vi "NEW_PRN Generation_Station1.vi"(8 "error in (no error)":errorcluster, 11 "Cluster in":T2) -> (0 "error out":errorcluster, 2 "cluster out":T2, 3 "QR CODE":string)   [LabVIEW 2017]
uses:
  <vilib>/addons/database/Connection.llb/Conn ObjectReference.ctl
  <vilib>/addons/database/NI_Database_API.lvlib
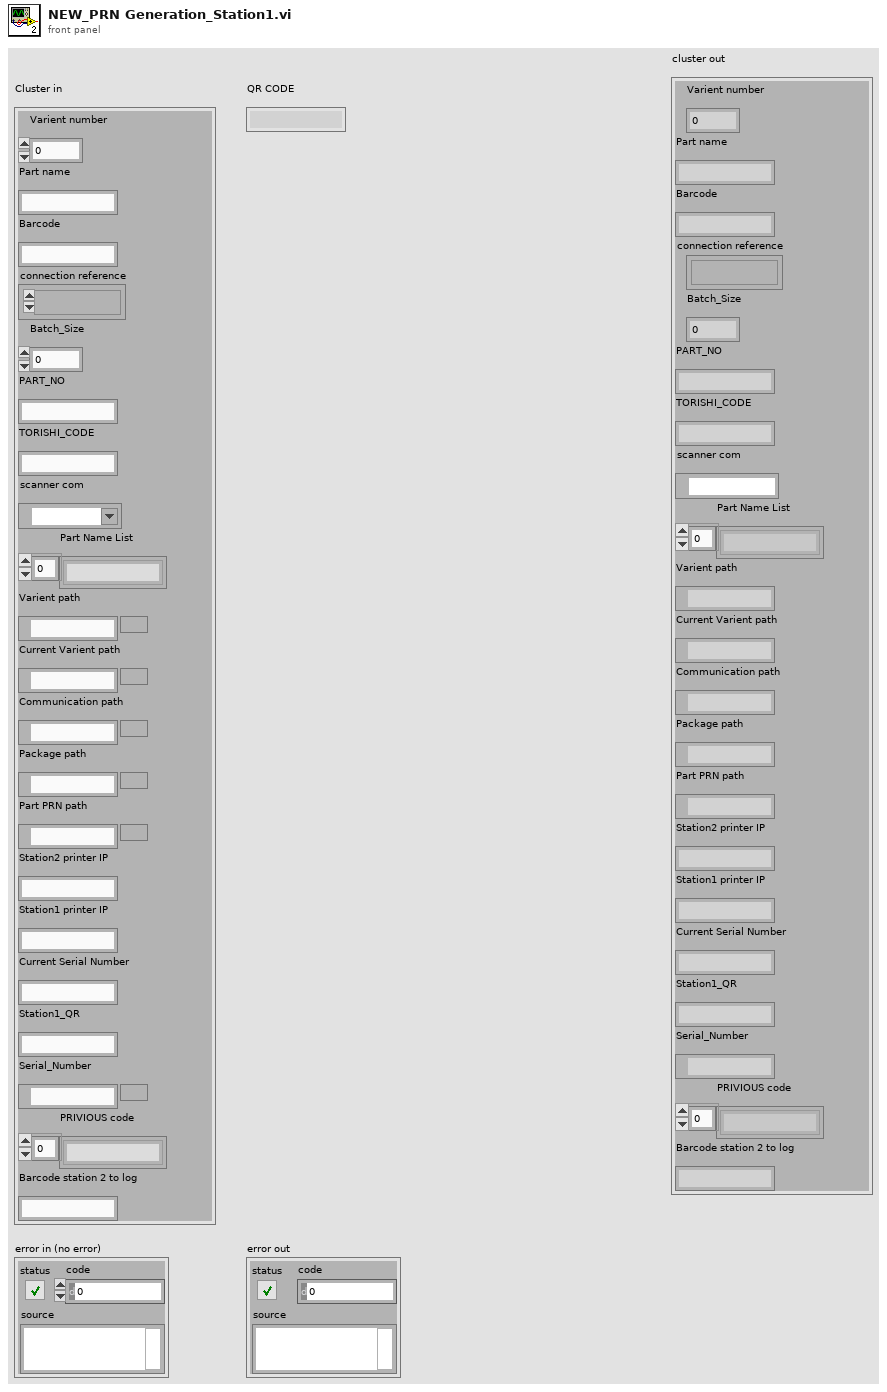
[diagram p1: front panel]
types:
  T1 = typedef "NI_Database_API.lvlib/Conn ObjectReference.ctl" = refnum<k1>
  T2 = cluster{"Varient number":u16, "Part name":string, "Barcode":string, "connection reference":T1, "Batch_Size":u16, "PART_NO":string, "TORISHI_CODE":string, "scanner com":refnum<visa-resource-name>, "Part Name List":string[], "Varient path":path, "Current Varient path":path, "Communication path":path, "Package path":path, "Part PRN path":path, "Station2 printer IP":string, "Station1 printer IP":string, "Current Serial Number":string, "Station1_QR":string, "Serial_Number":path, "PRIVIOUS code":string[], "Barcode station 2 to log":string}
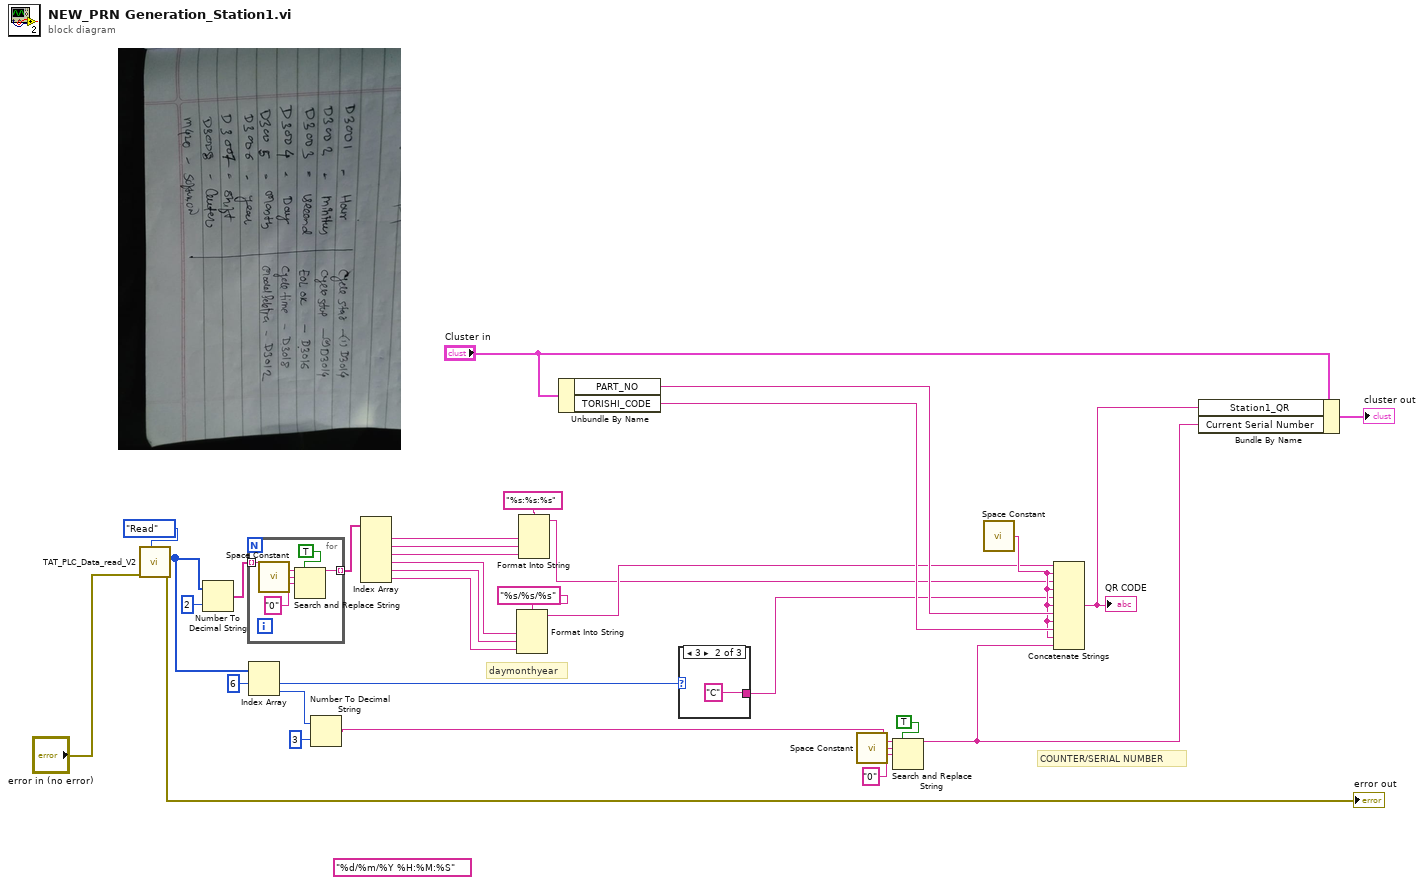
[diagram p0: block diagram]
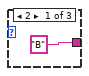
[diagram p2: hidden frame]
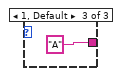
[diagram p3: hidden frame]
diagram:
  (unwired) "%d/%m/%Y %H:%M:%S" ("time format string (%c)")
  # "COUNTER/SERIAL NUMBER"
  # "daymonthyear"
  n1 = call "TAT_PLC_Data_read_V2.vi"("Enum"=enum16{"Read", "Write"}."Read", "error in (no error)"="error in (no error)") -> ("error out"=→"error out":errorcluster, "Array 2"=w7:u16[])  [unwired: 8 in]
  n2 = Number To Decimal String(number=w7, width (-)=i16 2) -> (decimal integer string=w2:string[])
  n3 = for {
    tunnel: w2 -> [w35] mode=indexing
    tunnel: [w34] -> w1 mode=indexing
    n4 = call <vilib>:"Space Constant.vi"() -> ("String"=w36:string)
    n5 = Search and Replace String(replace all?=TRUE ("replace all? (F)"), input string=w35, search string=w36, replace string="0" ("replace string (\"\")")) -> (result string=w34:string)  [unwired: 4 in, 3 out]
  }
  n6 = Index Array(array=w7, index #1=6 ("index")) -> (element #1=w5:u16, element #2=w4:u16)  [unwired: 1 in]
  n7 = Number To Decimal String(number=w4, width (-)=i16 3) -> (decimal integer string=w3:string)
  n8 = Index Array(array=w1) -> (element #1=w9:string, element #2=w18:string, element #3=w17:string, element #4=w29:string, element #5=w31:string, element #6=w30:string)  [unwired: 6 in]
  n9 = Format Into String(format string="%s/%s/%s" ("time format string (%c)"), w29, w31, w30) -> (resulting string=w16:string)  [unwired: 2 in, 1 out]
  n10 = Format Into String(format string="%s:%s:%s" ("time format string (%c)"), w9, w18, w17) -> (resulting string=w15:string)  [unwired: 2 in, 1 out]
  n11 = Unbundle By Name("Cluster in") -> ("PART_NO"=w25:string, "TORISHI_CODE"=w26:string)
  n12 = case shown="3" w5 {
    tunnel: ["B" "C" "A"] -> w14
    frame 2 {
    }
    frame 3 {
    }
    frame 1, Default {
    }
  }
  n13 = call <vilib>:"Space Constant.vi"() -> ("String"=w21:string)
  n14 = Search and Replace String(replace all?=TRUE ("replace all? (F)"), input string=w3, search string=w21, replace string="0" ("replace string (\"\")")) -> (result string=w12:string)  [unwired: 4 in, 3 out]
  n15 = call <vilib>:"Space Constant.vi"() -> ("String"=w20:string)
  n16 = Concatenate Strings(w16, w20, w15, w20, w14, w20, w25, w20, w26, w20, w12) -> (w10:string)
  "QR CODE" <- w10
  n17 = Bundle By Name(cluster="Cluster in", "Station1_QR"=w10, "Current Serial Number"=w12) -> (→"cluster out":T2)
